vi "IdleState.vi"(8 "error in (no error)":errorcluster, 9 "Cluster in":T2, 10 "Enum in":T1, 11 "Actual Start [i]":i64) -> (0 "error out":errorcluster, 2 "Cluster out":T2, 3 "Enum":T1)   [LabVIEW 2018]
uses:
  Type_Def Actuator Controls.ctl
  Type_Def_ControlState.ctl
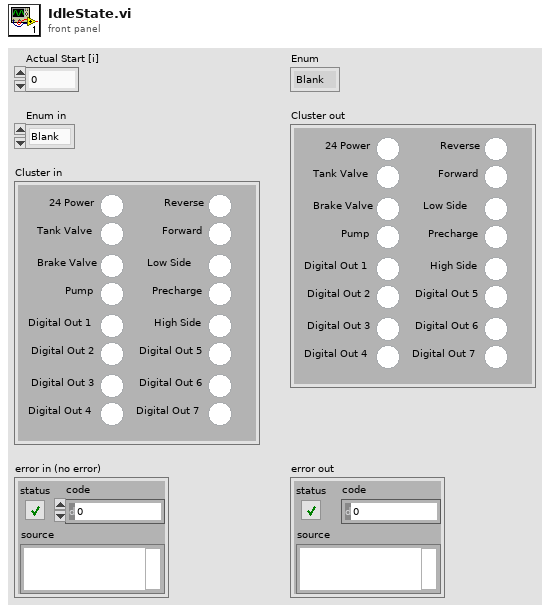
[diagram p1: front panel]
types:
  T1 = typedef "Type_Def_ControlState.ctl" = enum16{"Blank", "Systems Check", "Idle", "Ready", "Pushing", "CrawlingPrecharge", "Braking", "Fault", "Boot Up", "Unpowered", "Crawling", "Shutdown", "Service Push", "Service Wait", "Vent", "Precharge", "Cooldown"}
  T2 = typedef "Type_Def Actuator Controls.ctl" = cluster{"Reverse ":bool, "Forward":bool, "Low Side":bool, "Precharge":bool, "High Side":bool, "Digital Out 5":bool, "Digital Out 6":bool, "Digital Out 7 ":bool, "24 Power":bool, "Tank Valve ":bool, "Brake Valve":bool, "Pump":bool, "Digital Out 1 ":bool, "Digital Out 2":bool, "Digital Out 3":bool, "Digital Out 4 ":bool}
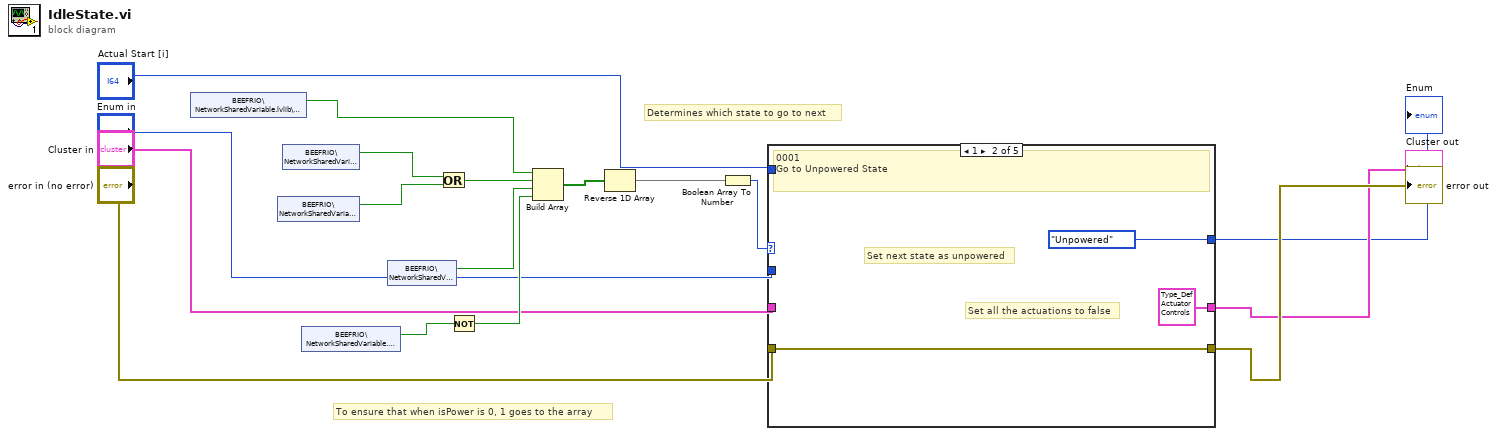
[diagram p0: block diagram]
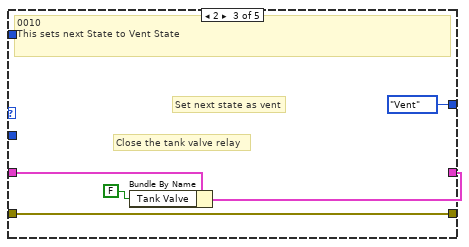
[diagram p3: hidden frame]
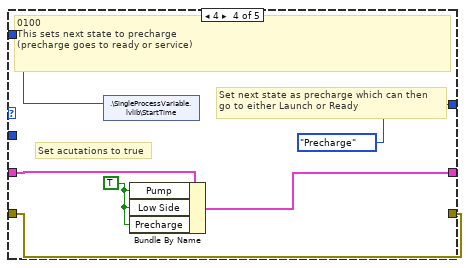
[diagram p4: hidden frame]
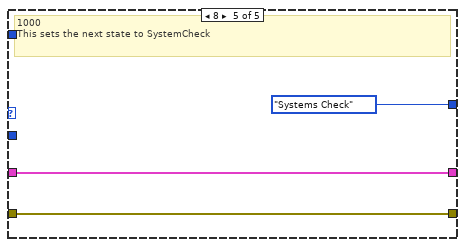
[diagram p5: hidden frame]
diagram:
  # "To ensure that when isPower is 0, 1 goes to the array"
  # "Determines which state to go to next"
  n1 = shared-variable "BEEFRIO\\NetworkSharedVariable.lvlib\\SystemCheck"() -> (w1:bool)  [unwired: 1 in, 1 out]
  n2 = shared-variable "BEEFRIO\\NetworkSharedVariable.lvlib\\Service"() -> (w12:bool)  [unwired: 1 in, 1 out]
  n3 = shared-variable "BEEFRIO\\NetworkSharedVariable.lvlib\\Ready"() -> (w13:bool)  [unwired: 1 in, 1 out]
  n4 = shared-variable "BEEFRIO\\NetworkSharedVariable.lvlib\\IsPowered"() -> (w10:bool)  [unwired: 1 in, 1 out]
  n5 = shared-variable "BEEFRIO\\NetworkSharedVariable.lvlib\\Vent"() -> (w6:bool)  [unwired: 1 in, 1 out]
  n6 = Or(x=w13, y=w12) -> (x .or. y?=w14:bool)
  n7 = Not(x=w10) -> (.not. x?=w11:bool)
  n8 = Build Array(w1, w14, w6, w11) -> (w7:bool[])
  n9 = Reverse 1D Array(array=w7) -> (reversed array=w8:bool[])
  n10 = Boolean Array To Number(Boolean array=w8) -> (number=w9:u32)
  n11 = case shown="1" w9 {
    tunnel: "Enum in" -> [w20 _ _ _ _]
    tunnel: [w20 Type_Def_ControlState."Unpowered" Type_Def_ControlState."Vent" Type_Def_ControlState."Precharge" Type_Def_ControlState."Systems Check"] -> w3
    tunnel: "Cluster in" -> [w19 _ w25 w33 w36]
    tunnel: [w19 T2 {"Reverse "=FALSE, "Forward"=FALSE, "Low Side"=FALSE, "Precharge"=FALSE, "High Side"=FALSE, "Digital Out 5"=FALSE, "Digital Out 6"=FALSE, "Digital Out 7 "=FALSE, "24 Power"=FALSE, "Tank Valve "=FALSE, "Brake Valve"=FALSE, "Pump"=FALSE, "Digital Out 1 "=FALSE, "Digital Out 2"=FALSE, "Digital Out 3"=FALSE, "Digital Out 4 "=FALSE} w26 w31 w36] -> w5
    tunnel: [w18 w21 w24 w30 w35] -> w15
    tunnel: "error in (no error)" -> [w18 w21 w24 w30 w35]
    tunnel: "Actual Start [i]" -> [_ _ _ w29 _]
    frame 0, Default {
      # "Does nothing and stays in Idle mode"
    }
    frame 1 {
      # "Set next state as unpowered"
      # "Set all the actuations to false"
      # "0001\nGo to Unpowered State"
    }
    frame 2 {
      # "Set next state as vent"
      # "Close the tank valve relay"
      # "0010\nThis sets next State to Vent State"
      n12 = Bundle By Name(cluster=w25, "Tank Valve"=FALSE) -> (w26:T2)
    }
    frame 4 {
      w32 = TRUE
      # "Set next state as precharge which can then \ngo to either Launch or Ready"
      # "Set acutations to true"
      # "0100\nThis sets next state to precharge \n(precharge goes to ready or service)"
      n13 = shared-variable ".\\SingleProcessVariable.lvlib\\StartTime"(w29) -> ()  [unwired: 1 in, 1 out]
      n14 = Bundle By Name(cluster=w33, "Pump"=w32, "Low Side"=w32, "Precharge"=w32) -> (w31:T2)
    }
    frame 8 {
      # "1000\nThis sets the next state to SystemCheck"
    }
  }
  "error out" <- w15
  "Cluster out" <- w5
  "Enum" <- w3
